vi "L1_Result_PhaseStep_Parsing.vi"() -> ()   [LabVIEW 2023]
uses:
  <vilib>/Utility/file.llb/Read Delimited Spreadsheet (string).vi
panel:
  in  "InPath":path=path "D:/_Project/_Code/LabVIEW/_CLC_Gen4/CLC_LV2023/CLC_Cali/SourceData/F22407150150_20250214-165216/F22407150150_20250214-165216_Result.csv"
  out "element":string
  in  "Test Item":u16(ring) items=["TX_H_Ch0_Freq26.5_In_Phase_Step", "TX_H_Ch0_Freq28_In_Phase_Step", "TX_H_Ch0_Freq29.5_In_Phase_Step", "TX_H_Ch0_Freq31_In_Phase_Step", "TX_H_Ch1_Freq26.5_In_Phase_Step", "TX_H_Ch1_Freq28_In_Phase_Step", "TX_H_Ch1_Freq29.5_In_Phase_Step", "TX_H_Ch1_Freq31_In_Phase_Step", "TX_H_Ch2_Freq26.5_In_Phase_Step", "TX_H_Ch2_Freq28_In_Phase_Step", "TX_H_Ch2_Freq29.5_In_Phase_Step", "TX_H_Ch2_Freq31_In_Phase_Step", "TX_H_Ch3_Freq26.5_In_Phase_Step", "TX_H_Ch3_Freq28_In_Phase_Step", "TX_H_Ch3_Freq29.5_In_Phase_Step", "TX_H_Ch3_Freq31_In_Phase_Step", "TX_V_Ch0_Freq26.5_In_Phase_Step", "TX_V_Ch0_Freq28_In_Phase_Step", "TX_V_Ch0_Freq29.5_In_Phase_Step", "TX_V_Ch0_Freq31_In_Phase_Step", "TX_V_Ch1_Freq26.5_In_Phase_Step", "TX_V_Ch1_Freq28_In_Phase_Step", "TX_V_Ch1_Freq29.5_In_Phase_Step", "TX_V_Ch1_Freq31_In_Phase_Step", "TX_V_Ch2_Freq26.5_In_Phase_Step", "TX_V_Ch2_Freq28_In_Phase_Step", "TX_V_Ch2_Freq29.5_In_Phase_Step", "TX_V_Ch2_Freq31_In_Phase_Step", "TX_V_Ch3_Freq26.5_In_Phase_Step", "TX_V_Ch3_Freq28_In_Phase_Step", "TX_V_Ch3_Freq29.5_In_Phase_Step", "TX_V_Ch3_Freq31_In_Phase_Step", "RX_H_Ch0_Freq26.5_In_Phase_Step", "RX_H_Ch0_Freq28_In_Phase_Step", "RX_H_Ch0_Freq29.5_In_Phase_Step", "RX_H_Ch0_Freq31_In_Phase_Step", "RX_H_Ch1_Freq26.5_In_Phase_Step", "RX_H_Ch1_Freq28_In_Phase_Step", "RX_H_Ch1_Freq29.5_In_Phase_Step", "RX_H_Ch1_Freq31_In_Phase_Step", "RX_H_Ch2_Freq26.5_In_Phase_Step", "RX_H_Ch2_Freq28_In_Phase_Step", "RX_H_Ch2_Freq29.5_In_Phase_Step", "RX_H_Ch2_Freq31_In_Phase_Step", "RX_H_Ch3_Freq26.5_In_Phase_Step", "RX_H_Ch3_Freq28_In_Phase_Step", "RX_H_Ch3_Freq29.5_In_Phase_Step", "RX_H_Ch3_Freq31_In_Phase_Step", "RX_V_Ch0_Freq26.5_In_Phase_Step", "RX_V_Ch0_Freq28_In_Phase_Step", "RX_V_Ch0_Freq29.5_In_Phase_Step", "RX_V_Ch0_Freq31_In_Phase_Step", "RX_V_Ch1_Freq26.5_In_Phase_Step", "RX_V_Ch1_Freq28_In_Phase_Step", "RX_V_Ch1_Freq29.5_In_Phase_Step", "RX_V_Ch1_Freq31_In_Phase_Step", "RX_V_Ch2_Freq26.5_In_Phase_Step", "RX_V_Ch2_Freq28_In_Phase_Step", "RX_V_Ch2_Freq29.5_In_Phase_Step", "RX_V_Ch2_Freq31_In_Phase_Step", "RX_V_Ch3_Freq26.5_In_Phase_Step", "RX_V_Ch3_Freq28_In_Phase_Step", "RX_V_Ch3_Freq29.5_In_Phase_Step", "RX_V_Ch3_Freq31_In_Phase_Step", "TX_H_com_gain_26.5GHz", "TX_V_com_gain_26.5GHz", "TX_H_com_gain_28GHz", "TX_V_com_gain_28GHz", "TX_H_com_gain_29.5GHz", "TX_V_com_gain_29.5GHz", "TX_H_com_gain_31GHz", "TX_V_com_gain_31GHz", "RX_H_com_gain_26.5GHz", "RX_V_com_gain_26.5GHz", "RX_H_com_gain_28GHz", "RX_V_com_gain_28GHz", "RX_H_com_gain_29.5GHz", "RX_V_com_gain_29.5GHz", "RX_H_com_gain_31GHz", "RX_V_com_gain_31GHz", "TX_H_all_gain_26.5GHz", "TX_V_all_gain_26.5GHz", "TX_H_all_gain_28GHz", "TX_V_all_gain_28GHz", "TX_H_all_gain_29.5GHz", "TX_V_all_gain_29.5GHz", "TX_H_all_gain_31GHz", "TX_V_all_gain_31GHz", "RX_H_all_gain_26.5GHz", "RX_V_all_gain_26.5GHz", "RX_H_all_gain_28GHz", "RX_V_all_gain_28GHz", "RX_H_all_gain_29.5GHz", "RX_V_all_gain_29.5GHz", "RX_H_all_gain_31GHz", "RX_V_all_gain_31GHz"]
  out "Data":string[](array[string])
  out "Item":string[](array[string])
  out "all rows":string[][](array[string])
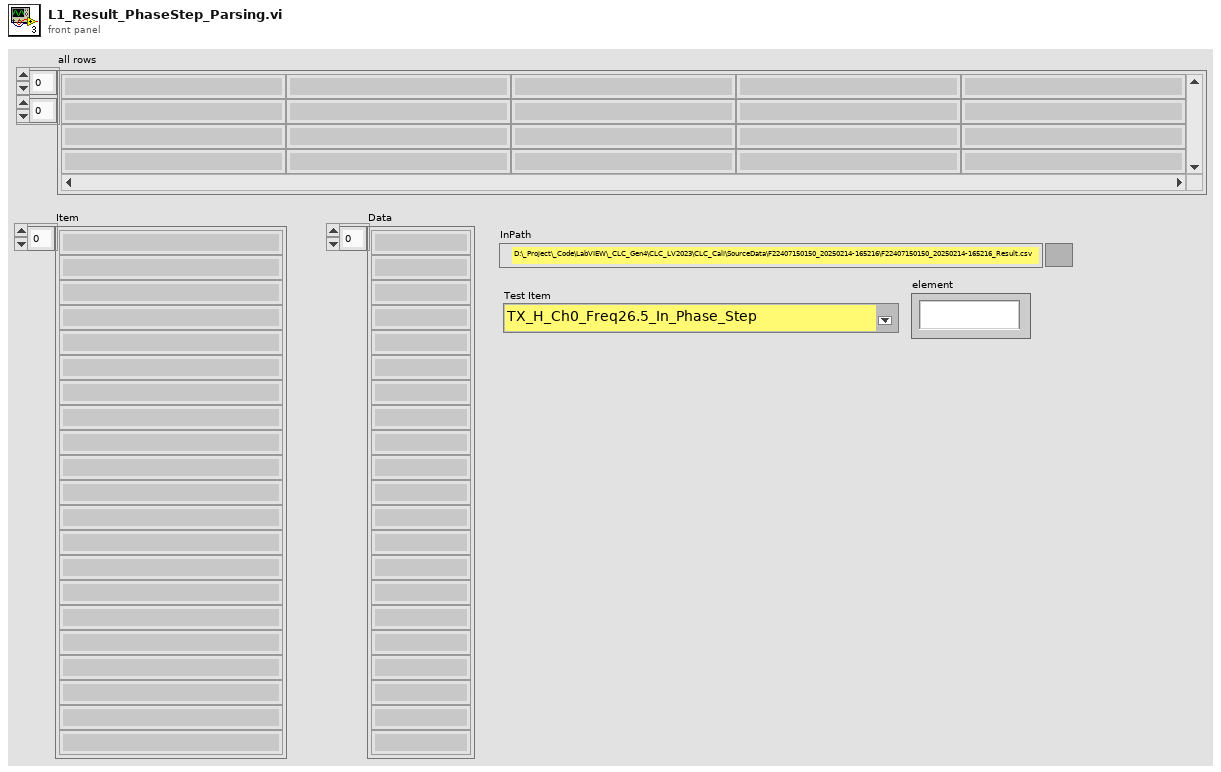
[diagram p1: front panel]
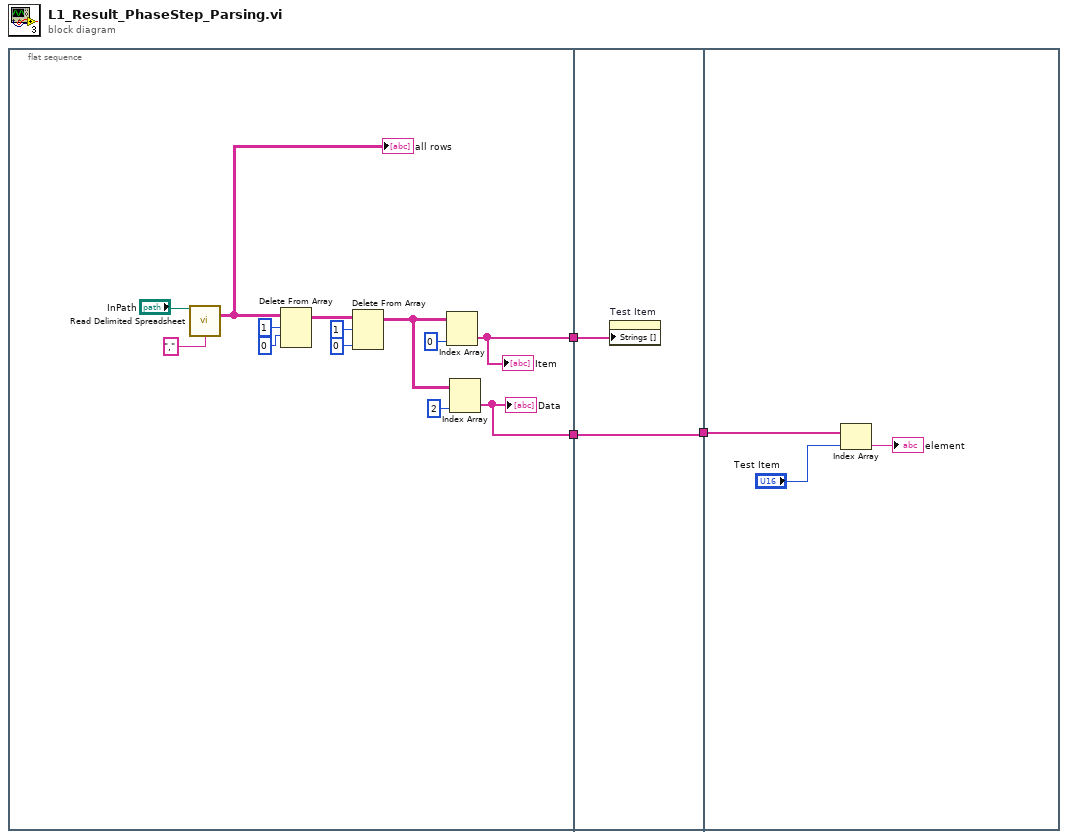
[diagram p0: block diagram]
diagram:
  n1 = flat-sequence {
    tunnel: [w5] -> w3
    tunnel: [w4] -> w2
    tunnel: w3 -> [w18]
    tunnel: w2 -> [w17]
    tunnel: [w17] -> w1
    tunnel: w1 -> [w21]
    frame #0 {
      n2 = call-poly <vilib>:"Read Delimited Spreadsheet.vi"("file path (dialog if empty)"="InPath", "delimiter (\\t)"="," ("delimiter (\\t)")) -> ("all rows"=w14:string[][])  [unwired: 8 in, 5 out]
      "all rows" <- w14
      n3 = Delete From Array(array=w14, length=1, index (row)=0) -> (array with subset deleted=w11:string[][])  [unwired: 1 in, 1 out]
      n4 = Delete From Array(array=w11, length=1, index (col)=0 ("disabled index (col)")) -> (array with subset deleted=w6:string[][])  [unwired: 1 in, 1 out]
      n5 = Index Array(array=w6, index (col)=0 ("disabled index (col)")) -> (element=w5:string[])  [unwired: 1 in]
      "Item" <- w5
      n6 = Index Array(array=w6, index (col)=2 ("disabled index (col)")) -> (element=w4:string[])  [unwired: 1 in]
      "Data" <- w4
    }
    frame #1 {
      n7 = property on="Test Item" class="Ring (strict)"("Strings []"=w18) -> ()  [unwired: 2 in, 2 out]
    }
    frame #2 {
      n8 = Index Array(array=w21, index="Test Item") -> (element=→"element":string)
    }
  }
